vi "FestoCPX.Global.vi"() -> ()   [LabVIEW 2016]
uses:
  FestoCPX.Data.Status.ctl
  FestoCPX.State.ctl
  FestoCPX.Data.Sets.ctl
  FestoCPX.DI.Sets.ctl
  FestoCPX.DI.ctl
  FestoCPX.DO.Sets.ctl
  FestoCPX.DO.ctl
panel:
  in  "FestoCPX.Sets":T1={"IP"="192.168.100.3", "Timeout_ms"=3000, "ReconnectPeriod_s"=5, "Config.DI"=[{"Name"="S.C. Emergency Stop", "Channel"=enum."0.0", "Negate"=FALSE}, {"Name"="S.C. Side Door Close", "Channel"=enum."0.1", "Negate"=FALSE}, {"Name"="S.C. Front Door Close", "Channel"=enum."0.2", "Negate"=FALSE}, {"Name"="S.C. Front Door Secured", "Channel"=enum."0.3", "Negate"=FALSE}, {"Name"="Button Start", "Channel"=enum."0.4", "Negate"=FALSE}, {"Name"="Button Stop", "Channel"=enum."0.5", "Negate"=FALSE}, {"Name"="Button Control", "Channel"=enum."0.6", "Negate"=FALSE}, {"Name"="Product Move Home", "Channel"=enum."1.0", "Negate"=FALSE}, {"Name"="Product Move Work", "Channel"=enum."1.1", "Negate"=FALSE}, {"Name"="Table Position", "Channel"=enum."1.2", "Negate"=FALSE}, {"Name"="Table Lock", "Channel"=enum."1.3", "Negate"=FALSE}, {"Name"="Product Lift A Home", "Channel"=enum."1.4", "Negate"=FALSE}, {"Name"="Product Lift B Home", "Channel"=enum."1.5", "Negate"=FALSE}, {"Name"="Product Arm OK", "Channel"=enum."1.6", "Negate"=FALSE}, {"Name"="Product Arm NOK", "Channel"=enum."1.7", "Negate"=FALSE}, {"Name"="Product Arm Work", "Channel"=enum."2.0", "Negate"=FALSE}, {"Name"="Revolver ID 1", "Channel"=enum."2.1", "Negate"=FALSE}, {"Name"="Revolver ID 2", "Channel"=enum."2.2", "Negate"=FALSE}, {"Name"="Revolver ID 3", "Channel"=enum."2.3", "Negate"=FALSE}, {"Name"="Revolver ID 4", "Channel"=enum."2.4", "Negate"=FALSE}, {"Name"="Revolver ID 5", "Channel"=enum."2.5", "Negate"=FALSE}, {"Name"="Air Pressure Inside", "Channel"=enum."2.6", "Negate"=FALSE}, {"Name"="Air Pressure Inlet", "Channel"=enum."2.7", "Negate"=FALSE}, {"Name"="Product Slot 1 A Present", "Channel"=enum."3.0", "Negate"=FALSE}, {"Name"="Product Slot 1 B Present", "Channel"=enum."3.1", "Negate"=FALSE}, {"Name"="Product Slot 2 A Present", "Channel"=enum."3.2", "Negate"=FALSE}, {"Name"="Product Slot 2 B Present", "Channel"=enum."3.3", "Negate"=FALSE}, {"Name"="Product Slot 3 A Present", "Channel"=enum."3.4", "Negate"=FALSE}, {"Name"="Product Slot 3 B Present", "Channel"=enum."3.5", "Negate"=FALSE}, {"Name"="Product Slot 4 A Present", "Channel"=enum."3.6", "Negate"=FALSE}, {"Name"="Product Slot 4 B Present", "Channel"=enum."3.7", "Negate"=FALSE}, {"Name"="Product Final A Present", "Channel"=enum."4.0", "Negate"=FALSE}, {"Name"="Product Final B Present", "Channel"=enum."4.1", "Negate"=FALSE}, {"Name"="Product Output A Present", "Channel"=enum."4.2", "Negate"=FALSE}, {"Name"="Product Output B Present", "Channel"=enum."4.3", "Negate"=FALSE}, {"Name"="Product Container OK Present", "Channel"=enum."4.4", "Negate"=FALSE}, {"Name"="Product Container NOK Present", "Channel"=enum."4.5", "Negate"=FALSE}], "Config.DO"=[{"Name"="Safety Reset", "Channel"=enum."4.0", "Negate"=FALSE, "Default"=FALSE}, {"Name"="Air Main Valve", "Channel"=enum."4.1", "Negate"=FALSE, "Default"=TRUE}, {"Name"="Door Lock", "Channel"=enum."4.2", "Negate"=FALSE, "Default"=FALSE}, {"Name"="Button LED Start", "Channel"=enum."4.3", "Negate"=FALSE, "Default"=FALSE}, {"Name"="Button LED Stop", "Channel"=enum."4.4", "Negate"=FALSE, "Default"=FALSE}, {"Name"="Button LED Control", "Channel"=enum."4.5", "Negate"=FALSE, "Default"=FALSE}, {"Name"="Traffic LED Red", "Channel"=enum."4.6", "Negate"=FALSE, "Default"=FALSE}, {"Name"="Traffic LED Orange", "Channel"=enum."4.7", "Negate"=FALSE, "Default"=FALSE}, {"Name"="Traffic LED Green", "Channel"=enum."5.0", "Negate"=FALSE, "Default"=FALSE}, {"Name"="Horn", "Channel"=enum."5.1", "Negate"=FALSE, "Default"=FALSE}, {"Name"="Laser Interlock", "Channel"=enum."5.2", "Negate"=FALSE, "Default"=FALSE}, {"Name"="Laser Trigger", "Channel"=enum."5.3", "Negate"=FALSE, "Default"=FALSE}, {"Name"="Laser Fume Extractor", "Channel"=enum."5.4", "Negate"=FALSE, "Default"=FALSE}, {"Name"="Product Suction Gripper Slot 1 A", "Channel"=enum."5.5", "Negate"=FALSE, "Default"=FALSE}, {"Name"="Product Suction Gripper Slot 1 B", "Channel"=enum."5.6", "Negate"=FALSE, "Default"=FALSE}, {"Name"="Product Suction Gripper Slot 2 A", "Channel"=enum."5.7", "Negate"=FALSE, "Default"=FALSE}, {"Name"="Product Suction Gripper Slot 2 B", "Channel"=enum."6.0", "Negate"=FALSE, "Default"=FALSE}, {"Name"="Product Suction Gripper Slot 3 A", "Channel"=enum."6.1", "Negate"=FALSE, "Default"=FALSE}, {"Name"="Product Suction Gripper Slot 3 B", "Channel"=enum."6.2", "Negate"=FALSE, "Default"=FALSE}, {"Name"="Product Suction Gripper Slot 4 A", "Channel"=enum."6.3", "Negate"=FALSE, "Default"=FALSE}, {"Name"="Product Suction Gripper Slot 4 B", "Channel"=enum."6.4", "Negate"=FALSE, "Default"=FALSE}, {"Name"="Product Suction Gripper Final A", "Channel"=enum."6.5", "Negate"=FALSE, "Default"=FALSE}, {"Name"="Product Suction Gripper Final B", "Channel"=enum."6.6", "Negate"=FALSE, "Default"=FALSE}, {"Name"="Lamp", "Channel"=enum."6.7", "Negate"=FALSE, "Default"=FALSE}, {"Name"="Q1 Product Move Work", "Channel"=enum."Q1K1", "Negate"=FALSE, "Default"=FALSE}, {"Name"="Q1 Product Move Home", "Channel"=enum."Q1K2", "Negate"=FALSE, "Default"=TRUE}, {"Name"="Q2 Table Turn Work", "Channel"=enum."Q2K1", "Negate"=FALSE, "Default"=FALSE}, {"Name"="Q2 Table Turn Home", "Channel"=enum."Q2K2", "Negate"=FALSE, "Default"=TRUE}, {"Name"="Q3 Product Lift A", "Channel"=enum."Q3K1", "Negate"=FALSE, "Default"=FALSE}, {"Name"="Q3 Product Lift B", "Channel"=enum."Q3K2", "Negate"=FALSE, "Default"=FALSE}, {"Name"="Q4 Product Arm OK", "Channel"=enum."Q4K1", "Negate"=FALSE, "Default"=FALSE}, {"Name"="Q4 Product Arm NOK", "Channel"=enum."Q4K2", "Negate"=FALSE, "Default"=FALSE}, {"Name"="Q5 Product Arm Work", "Channel"=enum."Q5K1", "Negate"=FALSE, "Default"=TRUE}]}
  out "FestoCPX.Abort":bool
  out "FestoCPX.Status":T6
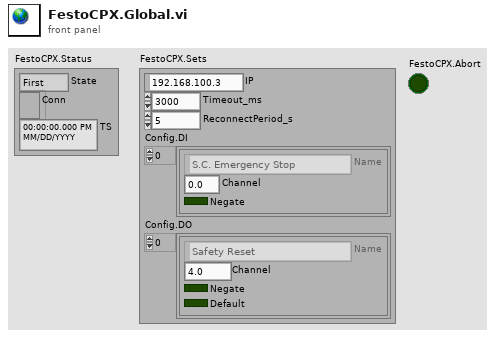
[diagram p1: front panel]
types:
  T1 = typedef "FestoCPX.Data.Sets.ctl" = cluster{"IP":string, "Timeout_ms":i32, "ReconnectPeriod_s":i32, "Config.DI":T2[], "Config.DO":T4[]}
  T2 = typedef "FestoCPX.DI.Sets.ctl" = cluster{"Name":string, "Channel":T3, "Negate":bool}
  T3 = typedef "FestoCPX.DI.ctl" = enum16{"0.0", "0.1", "0.2", "0.3", "0.4", "0.5", "0.6", "0.7", "1.0", "1.1", "1.2", "1.3", "1.4", "1.5", "1.6", "1.7", "2.0", "2.1", "2.2", "2.3", "2.4", "2.5", "2.6", "2.7", "3.0", "3.1", "3.2", "3.3", "3.4", "3.5", "3.6", "3.7", "4.0", "4.1", "4.2", "4.3", "4.4", "4.5", "4.6", "4.7"}
  T4 = typedef "FestoCPX.DO.Sets.ctl" = cluster{"Name":string, "Channel":T5, "Negate":bool, "Default":bool}
  T5 = typedef "FestoCPX.DO.ctl" = enum16{"4.0", "4.1", "4.2", "4.3", "4.4", "4.5", "4.6", "4.7", "5.0", "5.1", "5.2", "5.3", "5.4", "5.5", "5.6", "5.7", "6.0", "6.1", "6.2", "6.3", "6.4", "6.5", "6.6", "6.7", "Q1K1", "Q1K2", "Q2K1", "Q2K2", "Q3K1", "Q3K2", "Q4K1", "Q4K2", "Q5K1", "Q5K2", "Q6K1", "Q6K2"}
  T6 = typedef "FestoCPX.Data.Status.ctl" = cluster{"State":T7, "Conn":refnum<k5>, "TS":timestamp}
  T7 = typedef "FestoCPX.State.ctl" = enum16{"First", "Error", "Init", "Run"}
diagram:
